vi "AgNA_Save Sweep Trace.vi"(7 "Filename":string, 8 "Trace Data In":cluster{"Frequency":dbl[unit], "Power":dbl}[](array[cluster]), 9 "Test Stage":string, 10 "Frequency Range":cluster{"Min":dbl[unit], "Max":dbl[unit]} {"Max" format="%#.2g"; "Min" format="%#.2g"}, 11 "File Path":path) -> ()   [LabVIEW 2015]
uses:
  <vilib>/Utility/file.llb/Write To Spreadsheet File (string).vi
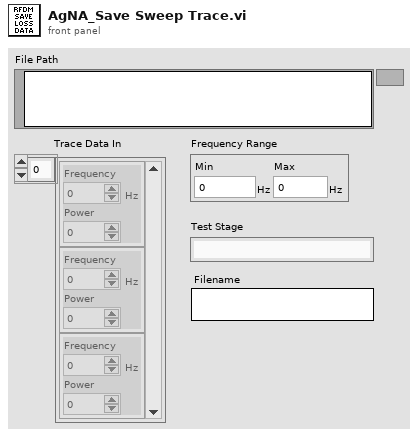
[diagram p1: front panel]
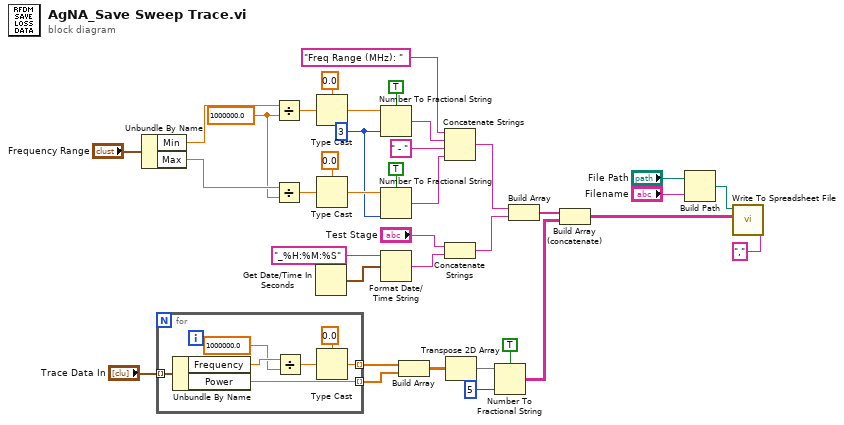
[diagram p0: block diagram]
diagram:
  w14 = 1000000.0
  w15 = i16 3 ("precision (6)")
  n1 = Unbundle By Name("Frequency Range") -> ("Min"=w22:dbl[unit], "Max"=w16:dbl[unit])
  n2 = for {
    tunnel: "Trace Data In" -> [w44] mode=indexing
    tunnel: [w43] -> w37 mode=indexing
    tunnel: [w41] -> w29 mode=indexing
    n3 = Unbundle By Name(w44) -> ("Frequency"=w39:dbl[unit], "Power"=w43:dbl)
    n4 = Divide(x=w39, y=1000000.0) -> (x/y=w40:dbl[unit])
    n5 = Type Cast(type=0.0, x=w40) -> (*(type *) &x=w41:dbl)
  }
  n6 = Divide(x=w22, y=w14) -> (x/y=w18:dbl[unit])
  n7 = Divide(x=w16, y=w14) -> (x/y=w17:dbl[unit])
  n8 = Get Date/Time In Seconds() -> (seconds since 1Jan1904=w6:timestamp)
  n9 = Type Cast(type=0.0, x=w18) -> (*(type *) &x=w20:dbl)
  n10 = Type Cast(type=0.0, x=w17) -> (*(type *) &x=w19:dbl)
  n11 = Number To Fractional String(use system decimal point (T)=TRUE, number=w20, precision (6)=w15) -> (F-format string=w13:string)  [unwired: 1 in]
  n12 = Number To Fractional String(use system decimal point (T)=TRUE, number=w19, precision (6)=w15) -> (F-format string=w12:string)  [unwired: 1 in]
  n13 = Format Date/Time String(time format string (%c)="_%H:%M:%S" ("string"), seconds (now)=w6) -> (date/time string=w4:string)  [unwired: 1 in]
  n14 = Build Array(w29, w37) -> (w33:dbl[][])
  n15 = Concatenate Strings("Freq Range (MHz): " ("string"), w13, " - " ("string"), w12) -> (w10:string)
  n16 = Concatenate Strings("Test Stage", w4) -> (w9:string)
  n17 = Transpose 2D Array(2D array=w33) -> (transposed array=w34:dbl[][])
  n18 = Number To Fractional String(use system decimal point (T)=TRUE, number=w34, precision (6)=i16 5) -> (F-format string=w32:string[][])  [unwired: 1 in]
  n19 = Build Array(w10, w9) -> (w28:string[])
  n20 = Build Array (concatenate)(w28, w32) -> (w31:string[][])
  n21 = Build Path(base path="File Path", name or relative path="Filename") -> (appended path=w1:path)
  n22 = call-poly <vilib>:"Write To Spreadsheet File.vi"("delimiter (\\t)"="," ("delimiter (\\t)"), "2D data"=w31, "file path (dialog if empty)"=w1) -> ()  [unwired: 5 in, 1 out]
